vi "Decode Crane Instruction.vi"(0 "Crane Instruction":string) -> (1 "From Stack":i32, 2 "#Crates to be moved":i32, 3 "To Stack":i32)   [LabVIEW 2020, in "AoC 2022.lvlib"]
uses:
  AoC 2022.lvlib
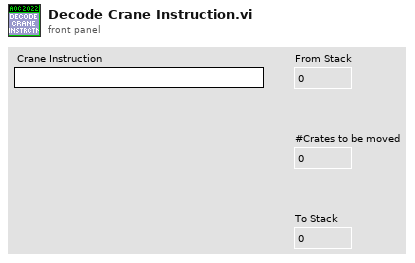
[diagram p1: front panel]
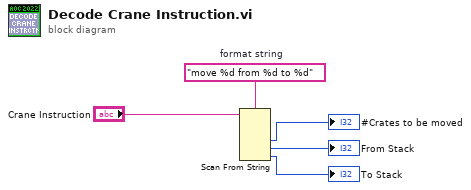
[diagram p0: block diagram]
diagram:
  w5 = "move %d from %d to %d"  # format string
  n1 = Scan From String(format string=w5, input string="Crane Instruction") -> (output 1=→"#Crates to be moved":i32, output 2=→"From Stack":i32, output 3=→"To Stack":i32)  [unwired: 5 in, 3 out]
